vi "VIS-IR_SringBlockTrig.vi"(8 "error in (no error)":errorcluster, 10 "channel 1, 2 or 3":u8=1, 11 "VIS-IR in":refnum<class "VIS-NIR.lvclass">) -> (0 "error out":errorcluster, 2 "Boolesch":bool, 3 "VIS-IR out":refnum<class "VIS-NIR.lvclass">)   [LabVIEW 2018, in "VIS-NIR.lvclass"]
uses:
  VIS-NIR.lvclass
  C:/Users/Sergey Denisov/Documents/REPS/TRANCON/Classes/Detector/Detector.lvclass
  Detector.lvclass/Detector.ctl
  Detector.lvclass
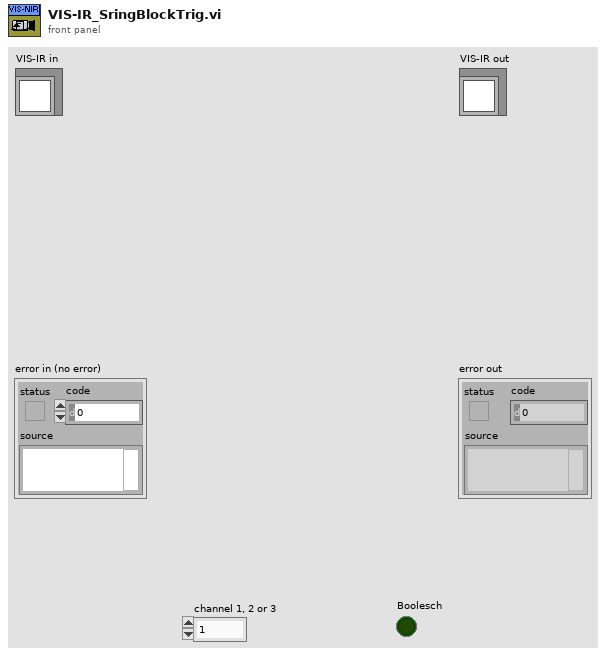
[diagram p1: front panel]
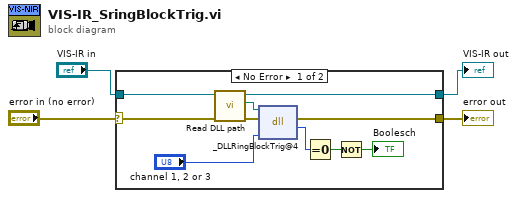
[diagram p0: block diagram]
diagram:
  n1 = case shown="No Error" "error in (no error)" {
    selector: "error in (no error)" -> [w14 w16]
    tunnel: [w10 w16] -> w3
    tunnel: [w6 w15] -> w1
    tunnel: "VIS-IR in" -> [w7 w15]
    frame No Error {
      n2 = call "Read DLL path.vi"("error in (no error)"=w14, "Detector in"=w7) -> ("error out"=w11:errorcluster, "DLL path"=w5:path, "Detector out"=w6:refnum<class "VIS-NIR.lvclass">)  [unwired: 7 in]
      n3 = dll-call lib="G:/SD/TRANCON/DLL/ESLSCDLL.dll" fn="_DLLRingBlockTrig@4" ("lwlscdll.dll:DLLTempGood")(path in=w5, error in=w11, "ch"="channel 1, 2 or 3") -> (error out=w10:errorcluster, "Rückgabetyp"=w9:u8)  [unwired: 2 in, 1 out]
      n4 = Equal To 0?(x=w9) -> (x = 0?=w13:bool)
      n5 = Not(x=w13) -> (.not. x?=→"Boolesch":bool)
    }
    frame Error {
    }
  }
  "error out" <- w3
  "VIS-IR out" <- w1
